vi "Autonomous Independent.vi"() -> ()   [LabVIEW 2016]
doc: "This VI is called when autonomous begins, and will automatically be terminated when autonomous ends. You can carry out timed or sensor driven robot movement independently without needing to return to the caller."
uses:
  <vilib>/Rock Robotics/Network Tables/NT Read Number.vi
  1_25_17/Action_type_def.ctl
panel:
  out "Defense Type":dbl=3.0
  in  "Auton_Modes":T2(array[cluster])=[{"Actions"=[{"Action"=enum."Drive", "Effort"=0.55, "Duration"=3.5}, {"Action"=enum."Nothing", "Effort"=0.0, "Duration"=0.0}]}, {"Actions"=[{"Action"=enum."Art Down", "Effort"=0.0, "Duration"=1.0}, {"Action"=enum."Drive", "Effort"=0.75, "Duration"=5.0}, {"Action"=enum."Art Up", "Effort"=0.0, "Duration"=1.0}]}, {"Actions"=[{"Action"=enum."Drive", "Effort"=1.0, "Duration"=3.0}, {"Action"=enum."Art Down", "Effort"=0.0, "Duration"=1.0}, {"Action"=enum."Drive", "Effort"=0.75, "Duration"=3.5}, {"Action"=enum."Art Up", "Effort"=0.0, "Duration"=1.0}]}, {"Actions"=[{"Action"=enum."Art Down", "Effort"=0.0, "Duration"=0.5}, {"Action"=enum."Drive", "Effort"=0.8, "Duration"=5.28}, {"Action"=enum."Art Up", "Effort"=0.0, "Duration"=1.0}, {"Action"=enum."Turn", "Effort"=-0.8, "Duration"=1.8}, {"Action"=enum."Nothing", "Effort"=0.0, "Duration"=0.1}, {"Action"=enum."Drive", "Effort"=0.8, "Duration"=1.75}, {"Action"=enum."Art Down", "Effort"=0.0, "Duration"=0.5}, {"Action"=enum."Vision Shot", "Effort"=0.0, "Duration"=4.0}]}, {"Actions"=[{"Action"=enum."Shift", "Effort"=0.0, "Duration"=0.0}, {"Action"=enum."Drive", "Effort"=1.0, "Duration"=0.1}, {"Action"=enum."Nothing", "Effort"=0.0, "Duration"=0.1}, {"Action"=enum."Drive", "Effort"=1.0, "Duration"=3.0}]}, {"Actions"=[{"Action"=enum."Shift", "Effort"=0.0, "Duration"=0.0}, {"Action"=enum."Drive", "Effort"=1.0, "Duration"=0.1}, {"Action"=enum."Nothing", "Effort"=0.0, "Duration"=0.1}, {"Action"=enum."Drive", "Effort"=1.0, "Duration"=3.0}]}, {"Actions"=[{"Action"=enum."Drive", "Effort"=0.55, "Duration"=4.0}, {"Action"=enum."Art Down", "Effort"=0.0, "Duration"=1.0}, {"Action"=enum."Drive", "Effort"=-0.5, "Duration"=0.6}, {"Action"=enum."Drive", "Effort"=0.75, "Duration"=1.0}, {"Action"=enum."Art Up", "Effort"=0.0, "Duration"=1.0}, {"Action"=enum."Drive", "Effort"=0.75, "Duration"=3.0}]}, {"Actions"=[{"Action"=enum."Art Down", "Effort"=0.0, "Duration"=0.5}, {"Action"=enum."Drive", "Effort"=0.55, "Duration"=4.25}, {"Action"=enum."Art Up", "Effort"=0.0, "Duration"=0.0}, {"Action"=enum."Nothing", "Effort"=0.0, "Duration"=0.3}, {"Action"=enum."Drive", "Effort"=0.9, "Duration"=2.0}]}, {"Actions"=[{"Action"=enum."Nothing", "Effort"=0.0, "Duration"=0.0}]}]
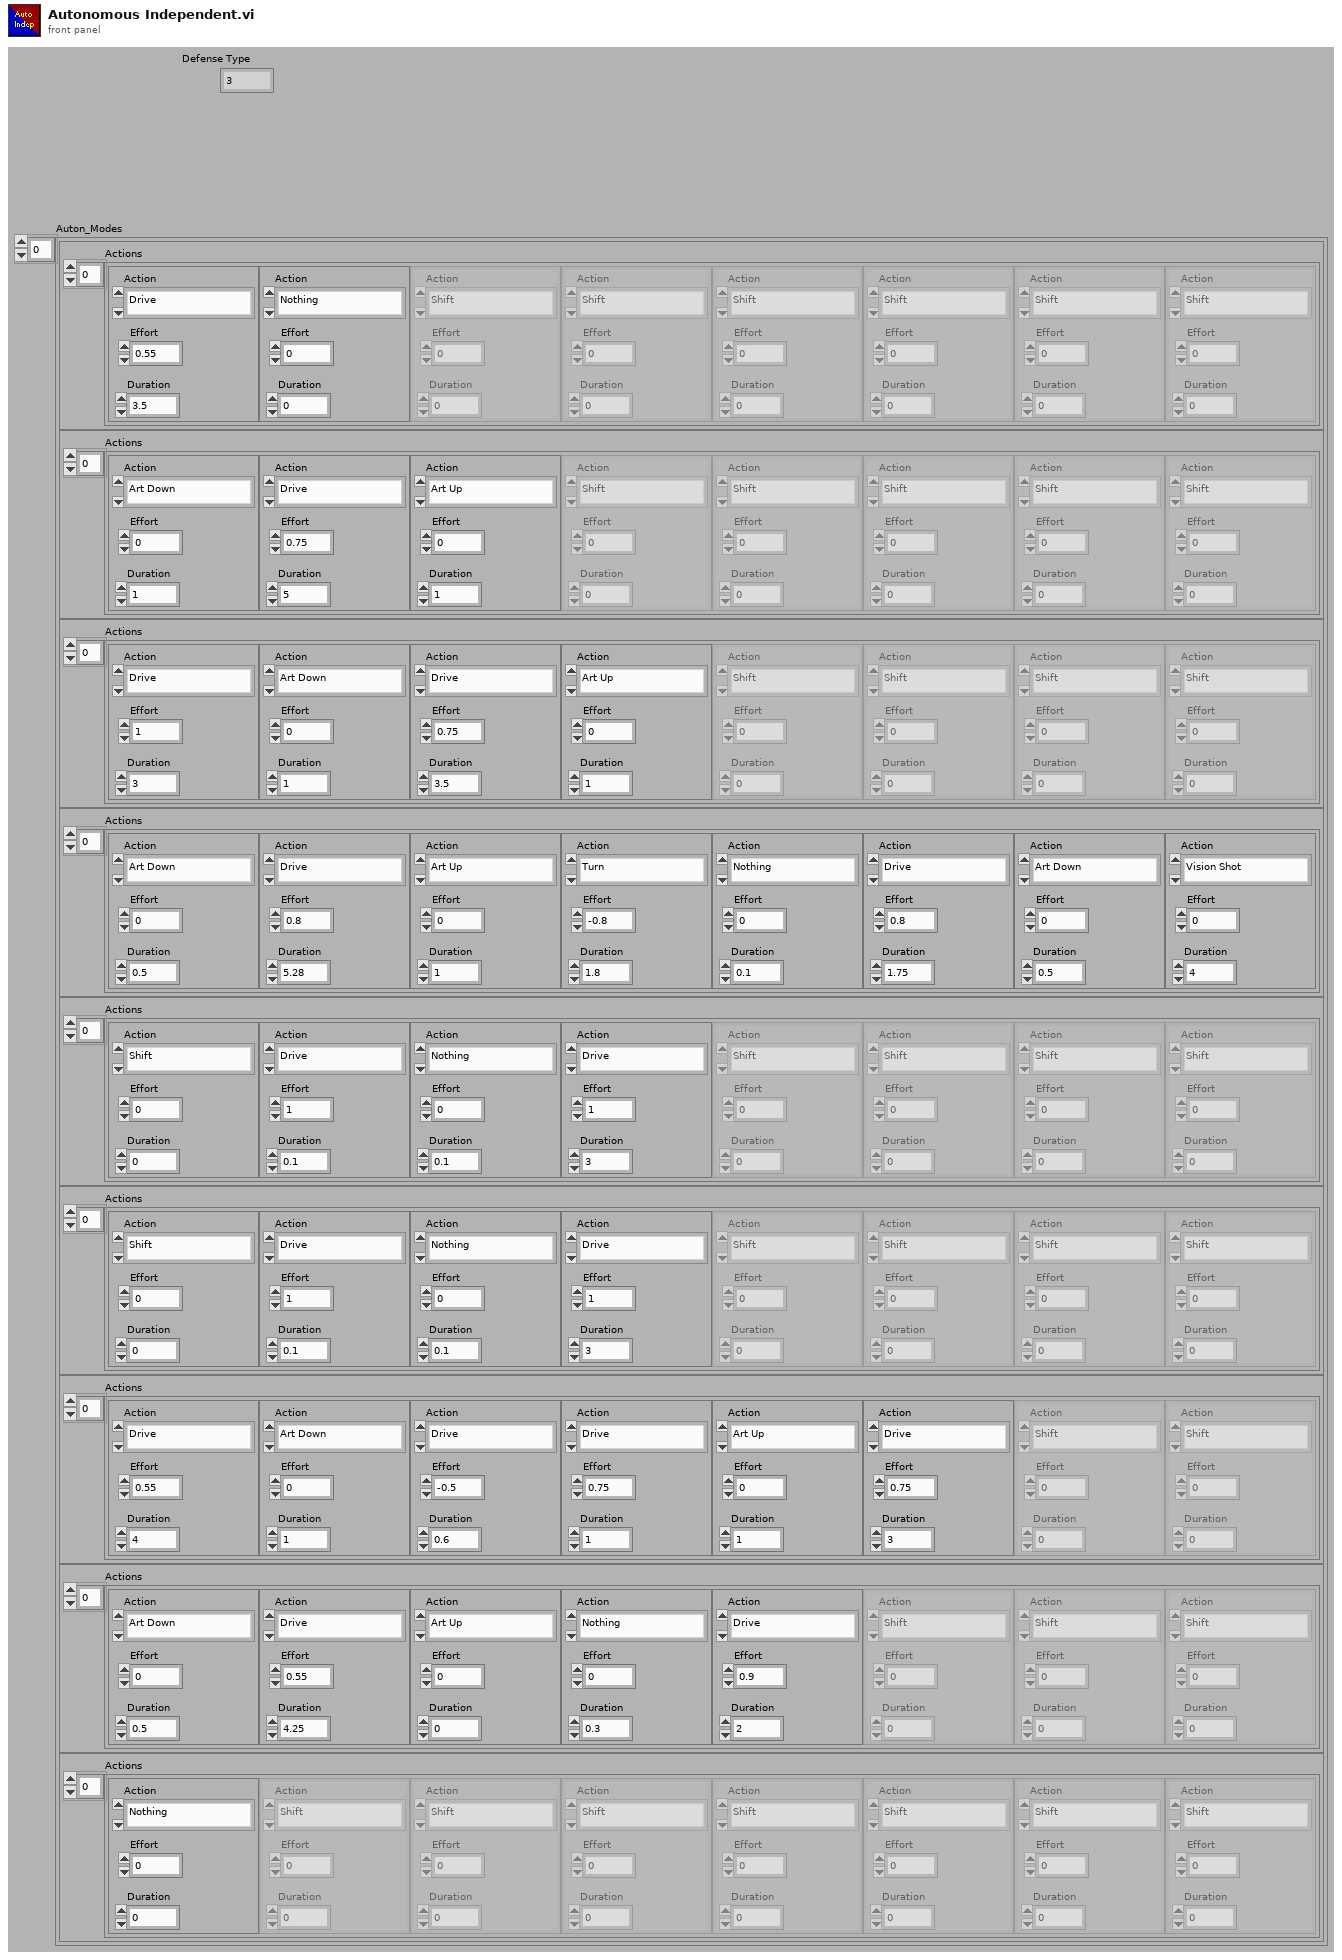
[diagram p1: front panel]
types:
  T1 = typedef "Action_type_def.ctl" = enum16{"Shift", "Shoot", "Move Articulates", "Nothing", "Drive", "Turn", "Vision Shot", "Art Up", "Art Down", "Test"}
  T2 = cluster{"Actions":cluster{"Action":T1, "Effort":dbl, "Duration":dbl}[]}[]
  T3 = cluster{"Actions":cluster{"Action":T1, "Effort":dbl, "Duration":dbl}[]}
  T4 = cluster{"Action":T1, "Effort":dbl, "Duration":dbl}[]
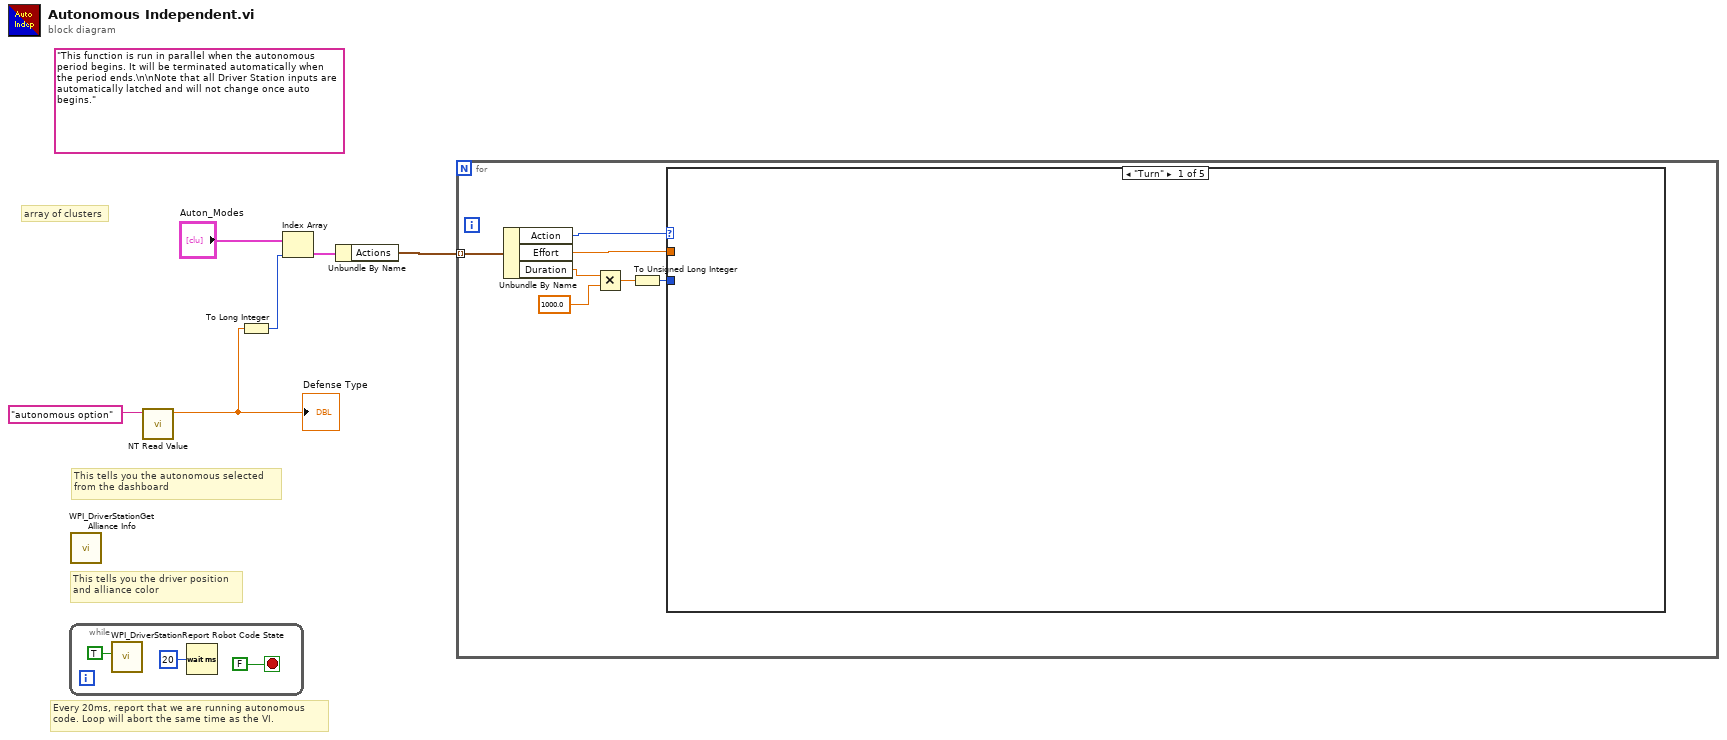
[diagram p0: block diagram]
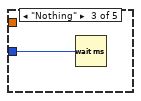
[diagram p3: hidden frame]
diagram:
  (unwired) "This function is run in parallel when the autonomous period begins. It will be terminated automatically when the period ends.\n\nNote that all Driver Station inputs are automatically latched and will not change once auto begins."
  # "This tells you the autonomous selected\nfrom the dashboard"
  # "array of clusters"
  # "Every 20ms, report that we are running autonomous\ncode. Loop will abort the same time as the VI."
  # "This tells you the driver position\nand alliance color"
  n1 = while {
    stop <- FALSE stop-if-true
    n2 = call <vilib>:"WPI_DriverStationReport Robot Code State.vi"("Autonomous"=TRUE) -> ()  [unwired: 10 in, 1 out]
    n3 = Wait (ms)(milliseconds to wait=u32 20) -> ()  [unwired: 1 out]
  }
  n4 = call <vilib>:"WPI_DriverStationGet Alliance Info.vi"() -> ()  [unwired: 12 out]
  n5 = call-poly <vilib>:"NT Read Value.vi"("Name"="autonomous option") -> ("Numeric"=w1:dbl)  [unwired: 9 in, 1 out]
  "Defense Type" <- w1
  n6 = To Long Integer(number=w1) -> (32bit integer=w3:i32)
  n7 = Index Array(array="Auton_Modes", index=w3) -> (element=w5:T3)
  n8 = Unbundle By Name(w5) -> ("Actions"=w6:T4)
  n9 = for {
    tunnel: w6 -> [w16] mode=indexing
    n10 = Unbundle By Name(w16) -> ("Action"=w15:T1, "Effort"=w14:dbl, "Duration"=w13:dbl)
    n11 = Multiply(x=w13, y=1000.0) -> (x*y=w10:dbl)
    n12 = To Unsigned Long Integer(number=w10) -> (unsigned 32bit integer=w11:u32)
    n13 = case shown="\"Turn\"" w15 {
      tunnel: w14 -> [_ _ _ _ _]
      tunnel: w11 -> [_ _ w17 _ _]
      frame "Turn" {
      }
      frame "Shift" {
      }
      frame "Nothing" {
        n14 = Wait (ms)(milliseconds to wait=w17) -> ()  [unwired: 1 out]
      }
      frame "Drive", Default {
      }
      frame "Shoot" {
      }
    }
  }
